vi "test_COM_trama.vi"() -> ()   [LabVIEW 2019]
uses:
  <vilib>/numeric/Random Number (Range) U64.vi
  <vilib>/numeric/sub_Random U32.vi
  <vilib>/Instr/_visa.llb/VISA Configure Serial Port (Instr).vi
panel:
  out "x = y?":bool
  out "bytes enviados":u32
  out "error out":errorcluster
  out "numero de tramas\ncorrectamente recibidas":i64
  out "trama enviada":string
  out "trama leida":string
  in  "stop":bool
  # "ESTE VI ES PARA PROBAR LA RUTINA DE ARDUINO DE LEER \nTRAMA DE DATOS EN STANDALONE GUARDADA EN LA CARPETA:\nC:\\Trabajo_Robot\\TFG_ROBOT\\CONTROL_ROBOT\\ARDUINO_TEST_ENVIOTRAMA"
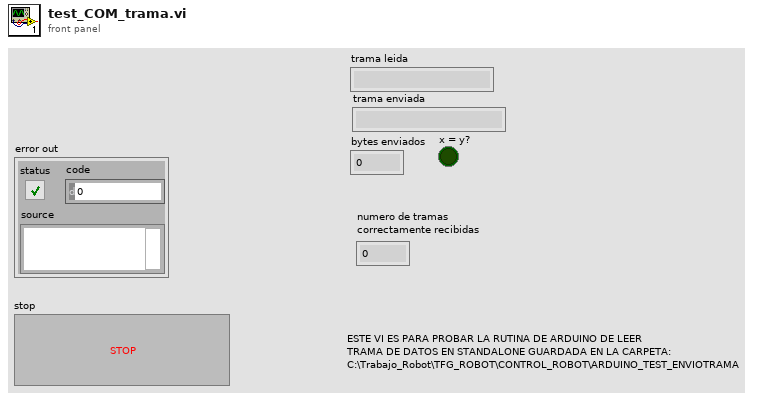
[diagram p1: front panel]
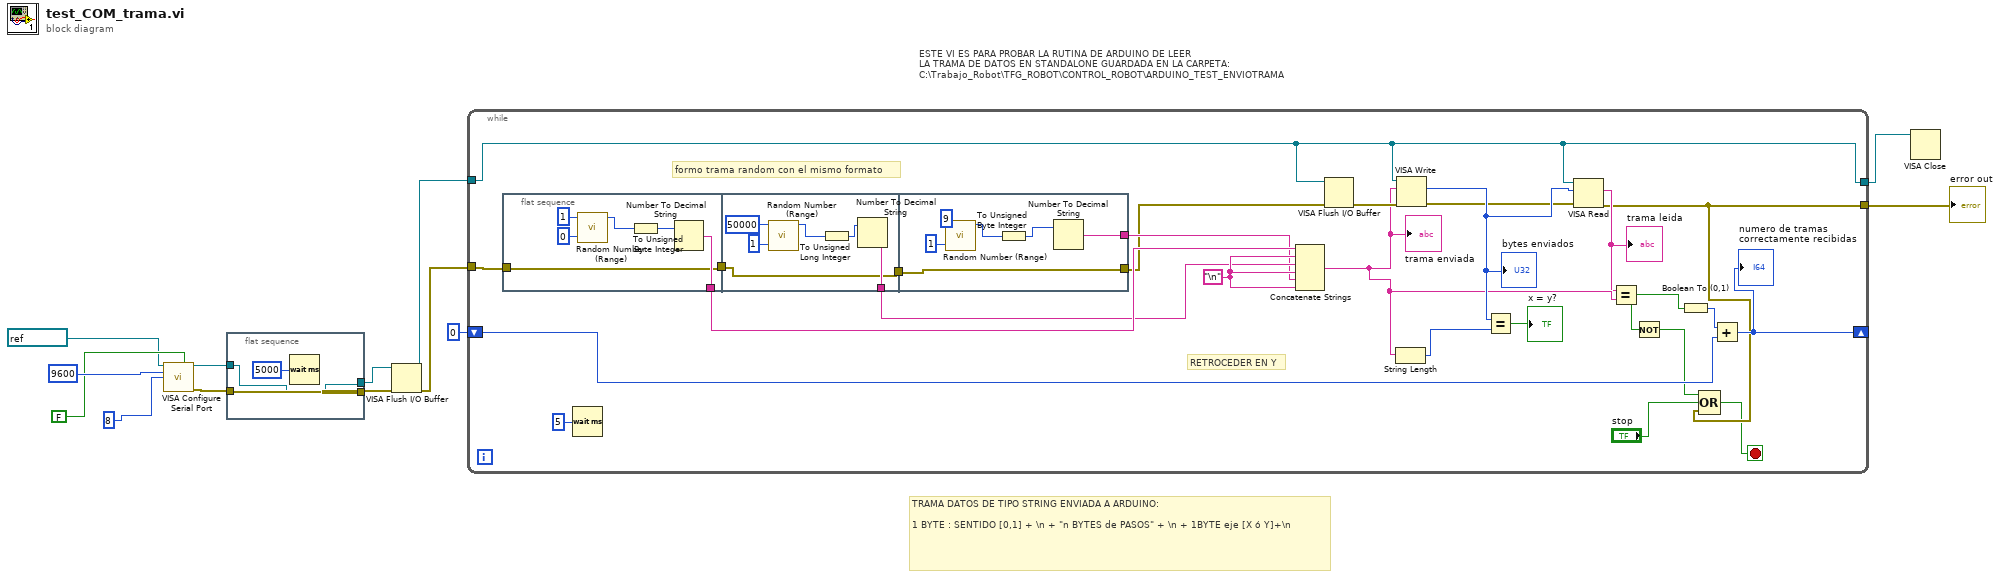
[diagram p0: block diagram]
diagram:
  # "TRAMA DATOS DE TIPO STRING ENVIADA A ARDUINO:\n\n1 BYTE : SENTIDO [0,1] + \\n + \"n BYTES de PASOS\" + \\n + 1BYTE eje [X ó Y]+\\n"
  # "ESTE VI ES PARA PROBAR LA RUTINA DE ARDUINO DE LEER \nLA TRAMA DE DATOS EN STANDALONE GUARDADA EN LA CARPETA:\nC:\\Trabajo_Robot\\TFG_ROBOT\\CONTROL_ROBOT\\ARDUINO_TEST_ENVIOTRAMA"
  n1 = call-poly "VISA Configure Serial Port"("VISA resource name"=refnum<visa-resource-name> "COM4", "Enable Termination\nChar (T)"=FALSE ("Enable Termination\nChar (T)"), "baud rate (9600)"=u32 9600, "data bits (8)"=u16 8) -> ("VISA resource name out"=w7:refnum<visa-resource-name>, "error out"=w11:errorcluster)  [unwired: 10 in]
  n2 = flat-sequence {
    tunnel: [w16] -> w8
    tunnel: w11 -> [w16]
    tunnel: [w14] -> w6
    tunnel: w7 -> [w14]
    frame #0 {
      n3 = Wait (ms)(milliseconds to wait=u32 5000) -> ()  [unwired: 1 out]
    }
  }
  n4 = VISA Flush I/O Buffer(VISA resource name=w6, error in (no error)=w8) -> (VISA resource name out=w4:refnum<visa-resource-name>, error out=w5:errorcluster)  [unwired: 1 in]
  n5 = while {
    tunnel: w5 -> [w24]
    tunnel: w4 -> [w17]
    tunnel: [w17] -> w1
    tunnel: [w27] -> w2
    shift-right: [w29] -> _
    shift-left: i16 0 -> [w30]
    stop <- w26 stop-if-true
    w40 = "\n"
    # "formo trama random con el mismo formato"
    # "RETROCEDER EN Y"
    n6 = flat-sequence {
      tunnel: [w43] -> w38
      tunnel: [w42] -> w25
      tunnel: w24 -> [w42]
      tunnel: [w50] -> w37
      tunnel: w25 -> [w48]
      tunnel: [w48] -> w23
      tunnel: [w55] -> w36
      tunnel: w23 -> [w54]
      tunnel: [w54] -> _
      tunnel: [w54] -> w22
      frame #0 {
        n7 = call-poly <vilib>:"Random Number (Range).vi"("lower bound (0)"=u64 0, "upper bound (100)"=u64 1) -> ("number"=w45:u64)  [unwired: 9 in]
        n8 = To Unsigned Byte Integer(number=w45) -> (unsigned 8bit integer=w44:u8)
        n9 = Number To Decimal String(number=w44) -> (decimal integer string=w43:string)  [unwired: 1 in]
      }
      frame #1 {
        n10 = call-poly <vilib>:"Random Number (Range).vi"("lower bound (0)"=u64 1, "upper bound (100)"=u64 50000) -> ("number"=w51:u64)  [unwired: 9 in]
        n11 = To Unsigned Long Integer(number=w51) -> (unsigned 32bit integer=w49:u32)
        n12 = Number To Decimal String(number=w49) -> (decimal integer string=w50:string)  [unwired: 1 in]
      }
      frame #2 {
        n13 = call-poly <vilib>:"Random Number (Range).vi"("lower bound (0)"=u64 1, "upper bound (100)"=u64 9) -> ("number"=w57:u64)  [unwired: 9 in]
        n14 = To Unsigned Byte Integer(number=w57) -> (unsigned 8bit integer=w56:u8)
        n15 = Number To Decimal String(number=w56) -> (decimal integer string=w55:string)  [unwired: 1 in]
      }
    }
    n16 = Wait (ms)(milliseconds to wait=u32 5) -> ()  [unwired: 1 out]
    n17 = Concatenate Strings(w38, w40, w37, w40, w36, w40) -> (w33:string)
    "trama enviada" <- w33
    n18 = VISA Flush I/O Buffer(VISA resource name=w17, error in (no error)=w22) -> (error out=w41:errorcluster)  [unwired: 1 in, 1 out]
    n19 = String Length(string=w33) -> (length=w39:i32)
    n20 = VISA Write(VISA resource name=w17, write buffer=w33, error in (no error)=w41) -> (return count=w35:u32, error out=w34:errorcluster)  [unwired: 1 out]
    "bytes enviados" <- w35
    n21 = Equal?(x=w35, y=w39) -> (x = y?=→"x = y?":bool)
    n22 = VISA Read(VISA resource name=w17, byte count=w35, error in (no error)=w34) -> (read buffer=w32:string, error out=w27:errorcluster)  [unwired: 2 out]
    "trama leida" <- w32
    n23 = Equal?(x=w32, y=w33) -> (x = y?=w19:bool)
    n24 = Not(x=w19) -> (.not. x?=w18:bool)
    n25 = Boolean To (0,1)(Boolean=w19) -> (0, 1=w31:i16)
    n26 = Compound Arithmetic op=OR(w18, "stop", w27) -> (w26:bool)
    n27 = Add(x=w31, y=w30) -> (x+y=w29:i16)
    "numero de tramas\ncorrectamente recibidas" <- w29
  }
  "error out" <- w2
  n28 = VISA Close(VISA resource name=w1) -> ()  [unwired: 1 in, 1 out]
